vi "Simple MsgPack Example.vi"() -> ()   [LabVIEW 2015, in "MsgPack.lvlib"]
uses:
  MsgPack.lvlib
  EncodeTypes/encodeInt32.vi
  EncodeTypes/encodeInt16.vi
  EncodeTypes/encodeInt8.vi
  SubVis/encodeFixedInt.vi
  DecodeTypes/decodeInt32.vi
panel:
  out "Variant Decode Error":errorcluster
  out "Decoded Number (Variant)":i32
  out "Decoded Number (Explict)":i32
  out "Explict Decode Error":errorcluster
  out "MsgPack (Encode Explict Type)":string
  out "Encode Error":errorcluster
  in  "Compress? (T)":bool=TRUE
  out "MsgPack (Encode Object)":string
  in  "Number":i32=12
  # "This Example VI shows two methods of Encoding MsgPack Packets.\n\nThe preferred way of using this library is to call \"encodeObject.vi\"\n     Note - You could use the function explictly if needed as shown.\n\n1- Enter a number and see the Corresponding MsgPack Packet.\n2- Change the Number Datatype and rerun to see the difference.\n\nNote - \"Compress? (T)\" is used to tell the Encoder how to process Integer values.\n    - True - Encoder compresses the actual integer value to smallest wire size datagram.  This is the MsgPack preferred method, because it produces the smallest total packet size.\n    - False - Encoder keeps the data type as is.  This permits preallocating arrays when sending arrays of INT/UINT values.  This decreases the encode time at the expense a larger packet size."
  # "This Example VI shows two methods of Decoding MsgPack Packets.\n\nThe preferred way of using this library is to call \"decodeObject.vi\".\n    Note - You could use the decode functions explictly if needed as shown, but care is needed to prevent decode errors.\n\nUsing the \"decodeObject.vi\" and \"Variant to Datatype\" allows for automatic type conversation.  This allows the encoder to use \"Compress?(T)\" to compress Integers to their smallest wire-size and then uncompress them without throwing errors.\n\nHint - Enter a small number and turn \"Compress? (T)\" on and off to see how the different ways of decoding will throw errors."
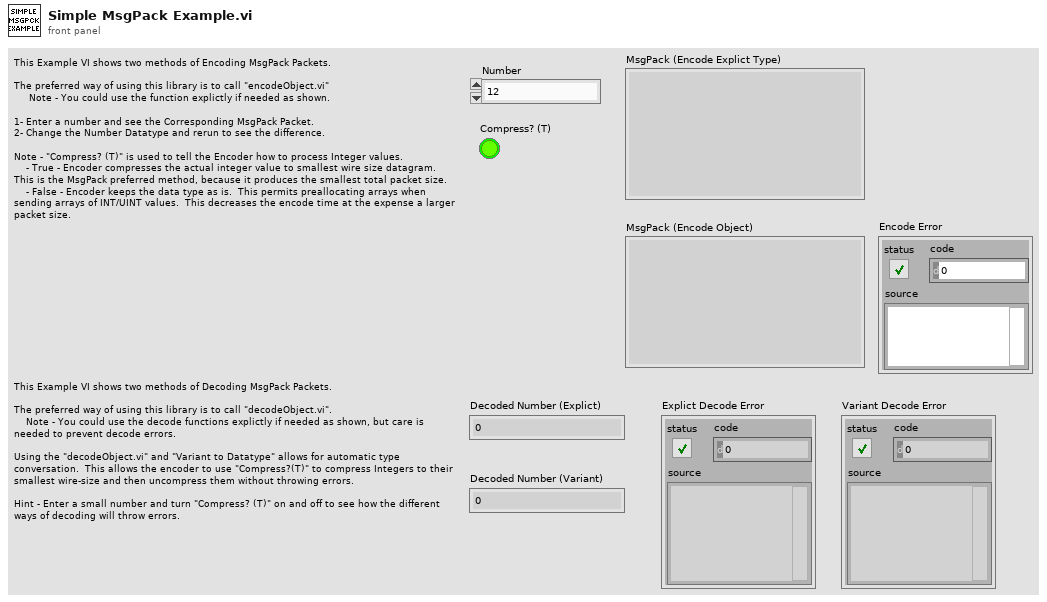
[diagram p1: front panel]
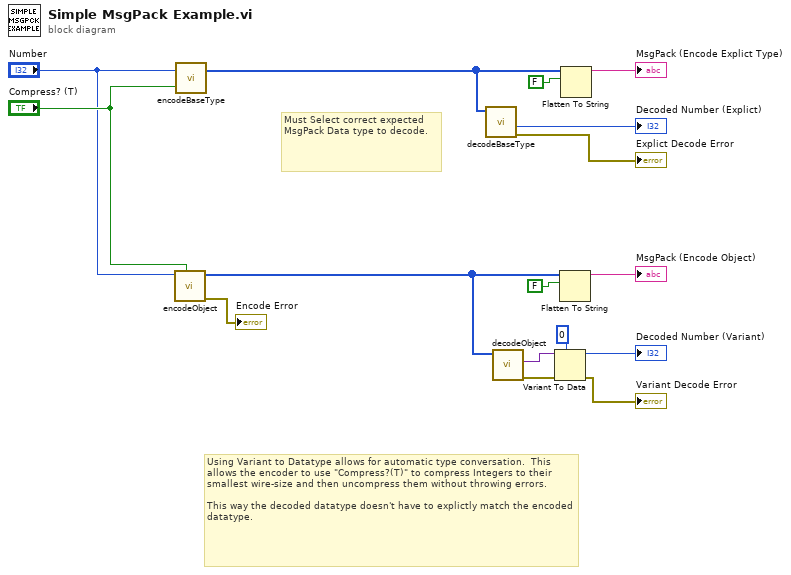
[diagram p0: block diagram]
diagram:
  # "Using Variant to Datatype allows for automatic type conversation.  This allows the encoder to use \"Compress?(T)\" to compress Integers to their smallest wire-size and then uncompress them without throwing errors.\n\nThis way the decoded datatype doesn't have to explictly match the encoded datatype."
  # "Must Select correct expected MsgPack Data type to decode."
  n1 = call "encodeObject.vi"("Compress? (T)"="Compress? (T)", "Variant"="Number") -> ("error out"=→"Encode Error":errorcluster, "MessagePack"=w6:u8[])  [unwired: 8 in]
  n2 = call-poly "encodeBaseType.vi"("Compress? (T)"="Compress? (T)", "Int32"="Number") -> ("MessagePack"=w9:u8[])  [unwired: 1 in]
  n3 = call-poly "decodeBaseType.vi"("ByteArray"=w9) -> ("error out"=→"Explict Decode Error":errorcluster, "Int32"=→"Decoded Number (Explict)":i32)  [unwired: 6 in, 3 out]
  n4 = call "decodeObject.vi"("ByteArray"=w6) -> ("error out"=w5:errorcluster, "Variant"=w3:variant)  [unwired: 7 in, 2 out]
  n5 = Variant To Data(error in=w5, type=0, Variant=w3) -> (data=→"Decoded Number (Variant)":i32, error out=→"Variant Decode Error":errorcluster)
  n6 = Flatten To String(anything=w6, prepend array or string size? (T)=FALSE) -> (data string=→"MsgPack (Encode Object)":string)  [unwired: 2 in, 2 out]
  n7 = Flatten To String(anything=w9, prepend array or string size? (T)=FALSE) -> (data string=→"MsgPack (Encode Explict Type)":string)  [unwired: 2 in, 2 out]
